vi "BCU诊断标定.vi"(8 "CAN端口":u16(ring) items=["0", "1"], 9 "设备索引号":u16(ring) items=["0", "1", "2", "3", "4", "5", "6", "7", "8", "9", "10", "11", "12", "13", "14", "15", ""], 10 "CAN卡类型":u32(ring)=21 items=["PCI5121"=1, "PCI9810"=2, "USBCAN1"=3, "USBCAN2"=4, "PCI9820"=5, "PCI5110"=7, "CANLite(mini)"=8, "ISA9620"=9, "ISA5420"=10, "PC104CAN"=11, "DNP9810"=13, "PCI9840B"=14, "PC104C2"=15, "PCI9820I"=16, "pec9920"=18, "USBCAN_E_U"=20, "USBCAN_2E_U"=21], 11 "Myindex":dbl=1.0) -> (3 "成功":bool)   [LabVIEW 2013]
uses:
  <vilib>/Utility/config.llb/Read Key (String).vi
  <vilib>/Utility/config.llb/Write Key (Path).vi
  <vilib>/Utility/file.llb/Write To Spreadsheet File (string).vi
  <vilib>/Utility/config.llb/Write Key (String).vi
  <vilib>/Utility/config.llb/NI_LVConfig.lvlib
  <vilib>/Utility/file.llb/Read From Spreadsheet File (string).vi
panel:
  out "读取超时":bool
  out "流控帧":bool
  out "流控帧 2":bool=TRUE
  in  "二维码 2":string="BNET01"
  out "失败?":bool=TRUE
  in  "主板选项":string(tree)="项目信息"
  out "重试次数":u8
  in  "模块版本读取":bool
  in  "模块软件版本":T1(ring)
  out "模块软件版本 2":i32(listbox)=-1
  out "从板信息":T2
  out "从板项目信息":bool
  out "项目信息结果":bool
  out "正级继电器 10":bool
  out "正级继电器 9":bool
  out "正级继电器 8":bool
  out "正级继电器 7":bool
  out "正级继电器 6":bool
  out "正级继电器 5":bool
  out "正级继电器 4":bool
  out "正级继电器 3":bool
  out "正级继电器 2":bool
  out "正级继电器 12":bool
  out "正级继电器 11":bool
  in  "DO1 2":bool
  out "模块个数":u8[](array[numeric])
  out "模块版本值":string[][](array[string])
  out "模块版本名称":string[][](array[string])
  out "硬件版本":string[](array[string])
  out "项目软件版本":string[](array[string])
  out "平台软件版本":string[](array[string])
  in  "读参数":T3
  out "MODEL号":u8[](array[numeric])
  out "主板数据":T4
  in  "布尔":bool=TRUE
  out "1 13":bool
  in  "error out":errorcluster
  out "key names":string[](array[string])
  out "输出数组":string[][](array[string])
  in  "当前从板板号":u8=1
  in  "高压参数":T5={"充电能量阀值"=375.0, "放电能量阀值"=375.0, "电流增益"=0.0, "平均电流"=0.0, "电压增益"=0.0, "平均电压"=0.0}
  in  "清BUFF":bool=TRUE
  out "继电器超时处理":bool
  in  "判定3":bool=TRUE
  out "判定2":bool
  in  "消除":bool
  in  "控制1":bool
  out "命令序号":u8=5
  in  "停止 2":bool
  in  "停止":bool
  in  "选项卡控件":enum32{"主板", "从板"}(tab)=enum."从板"
  in  "主板数据":string[][](table)=[["参数", "写入", "读取", "参数", "写入", "读取", "一级故障", "写入", "读取", "二级故障", "写入", "读取", "三张故障", "写入", "读取", "参数", "写入", "读取", "电池信息", "写入", "读取", "历史信息", "写入", "读取"], ["", "", "", "humd_sensr_no", "", "", "总电压过高", "", "", "总电压过高", "", "", "总电压过高", "", "", "风机开启温度", "", "", "电池串联数", "", "", "历史最高电压", "", ""], ["", "", "", "温度传感器类型", "", "", "总电压过低", "", "", "总电压过低", "", "", "总电压过低", "", "", "风机关闭温度", "", "", "电池并联数", "", "", "历史最低电压", "", ""], ["", "", "", "电流传感器类型", "", "", "温度过高", "", "", "温度过高", "", "", "温度过高", "", "", "加热开启温度", "", "", "电池厂商", "", "", "历史电池电压极差", "", ""], ["", "", "", "集成单板电压个数", "", "", "温度过低", "", "", "温度过低", "", "", "温度过低", "", "", "加热关闭温度", "", "", "电池类型", "", "", "历史最高平均电压", "", ""], ["", "", "", "集成单体温度个数", "", "", "整组温度不均衡", "", "", "整组温度不均衡", "", "", "整组温度不均衡", "", "", "风机开启温差", "", "", "年", "", "", "历史最低平均电压", "", ""], ["", "", "", "SOC", "", "", "单组电压不均衡", "", "", "单组电压不均衡", "", "", "单组电压不均衡", "", "", "风机关闭温差", "", "", "月", "", "", "历史最高端电压", "", ""], ["", "", "", "电池额定容量", "", "", "整组电压不均衡", "", "", "整组电压不均衡", "", "", "整组电压不均衡", "", "", "最大允许单体电压", "", "", "日", "", "", "历史最低端电压", "", ""], ["", "", "", "电池实际容量", "", "", "单体电压过高", "", "", "单体电压过高", "", "", "单体电压过高", "", "", "最大允许总电压", "", "", "电池包额定能量", "", "", "历史最高温度", "", ""], ["", "", "", "配置文件版本", "", "", "单体电压过低", "", "", "单体电压过低", "", "", "单体电压过低", "", "", "最大允许充电电流", "", "", "电池包额定容量", "", "", "历史最低温度", "", ""], ["", "", "", "车牌号", "", "", "充电电流过高", "", "", "充电电流过高", "", "", "充电电流过高", "", "", "最大允许温度", "", "", "电池包额定总电压", "", "", "历史电池温度极差", "", ""], ["", "", "", "从板板号", "", "", "放电电流过高", "", "", "放电电流过高", "", "", "放电电流过高", "", "", "最小充电电流", "", "", "电池包组号", "", "", "历史最高平均温度", "", ""], ["", "", "", "SOH", "", "", "单组温度不均衡", "", "", "单组温度不均衡", "", "", "单组温度不均衡", "", "", "电流步长", "", "", "电池包产权标识", "", "", "历史最低平均温度", "", ""], ["", "", "", "SOE", "", "", "SOC过高", "", "", "SOC过高", "", "", "SOC过高", "", "", "最小允许单体电压", "", "", "电池包应用车型", "", "", "平均温度分布", "", ""], ["", "", "", "产品编号", "", "", "SOC过低", "", "", "SOC过低", "", "", "SOC过低", "", "", "最大允许充电温度", "", "", "正极接触器寿命", "", "", "最低温度分布", "", ""], ["", "", "", "", "", "", "", "", "", "", "", "", "", "", "", "最小允许温度", "", "", "负极接触器寿命", "", "", "最高温度分布", "", ""], ["", "", "", "", "", "", "", "", "", "", "", "", "", "", "", "充电时间", "", "", "预充电接触器寿命", "", "", "最大极差温度分布", "", ""], ["", "", "", "", "", "", "", "", "", "", "", "", "", "", "", "", "", "", "充电接触器寿命", "", "", "历史最大充电功率", "", ""], ["", "", "", "", "", "", "", "", "", "", "", "", "", "", "", "", "", "", "车辆VIN号", "", "", "历史最大放电功率", "", ""], ["", "", "", "", "", "", "", "", "", "", "", "", "", "", "", "", "", "", "电池放空次数", "", "", "历史最大充电电流", "", ""], ["", "", "", "", "", "", "", "", "", "", "", "", "", "", "", "", "", "", "充满次数", "", "", "历史最大放电电流", "", ""], ["", "", "", "", "", "", "", "", "", "", "", "", "", "", "", "", "", "", "充电次数", "", "", "电池组工作电流分布", "", ""], ["", "", "", "", "", "", "", "", "", "", "", "", "", "", "", "", "", "", "", "", "", "电池组SOC分布", "", ""], ["", "", "", "", "", "", "", "", "", "", "", "", "", "", "", "", "", "", "", "", "", "电池总充电安时", "", ""], ["", "", "", "", "", "", "", "", "", "", "", "", "", "", "", "", "", "", "", "", "", "电池总放电安时", "", ""], ["", "", "", "", "", "", "", "", "", "", "", "", "", "", "", "", "", "", "", "", "", "电池剩余容量", "", ""], ["", "", "", "", "", "", "", "", "", "", "", "", "", "", "", "", "", "", "", "", "", "", "", ""], ["", "", "", "", "", "", "", "", "", "", "", "", "", "", "", "", "", "", "", "", "", "", "", ""], ["", "", "", "", "", "", "", "", "", "", "", "", "", "", "", "", "", "", "", "", "", "", "", ""], ["", "", "", "", "", "", "", "", "", "", "", "", "", "", "", "", "", "", "", "", "", "", "", ""], ["", "", "", "", "", "", "", "", "", "", "", "", "", "", "", "", "", "", "", "", "", "", "", ""], ["", "", "", "", "", "", "", "", "", "", "", "", "", "", "", "", "", "", "", "", "", "", "", ""], ["", "", "", "", "", "", "", "", "", "", "", "", "", "", "", "", "", "", "", "", "", "", "", ""], ["", "", "", "", "", "", "", "", "", "", "", "", "", "", "", "", "", "", "", "", "", "", "", ""], ["", "", "", "", "", "", "", "", "", "", "", "", "", "", "", "", "", "", "", "", "", "", "", ""], ["", "", "", "", "", "", "", "", "", "", "", "", "", "", "", "", "", "", "", "", "", "", "", ""], ["", "", "", "", "", "", "", "", "", "", "", "", "", "", "", "", "", "", "", "", "", "", "", ""], ["", "", "", "", "", "", "", "", "", "", "", "", "", "", "", "", "", "", "", "", "", "", "", ""], ["", "", "", "", "", "", "", "", "", "", "", "", "", "", "", "", "", "", "", "", "", "", "", ""], ["", "", "", "", "", "", "", "", "", "", "", "", "", "", "", "", "", "", "", "", "", "", "", ""], ["", "", "", "", "", "", "", "", "", "", "", "", "", "", "", "", "", "", "", "", "", "", "", ""], ["", "", "", "", "", "", "", "", "", "", "", "", "", "", "", "", "", "", "", "", "", "", "", ""], ["", "", "", "", "", "", "", "", "", "", "", "", "", "", "", "", "", "", "", "", "", "", "", ""], ["", "", "", "", "", "", "", "", "", "", "", "", "", "", "", "", "", "", "", "", "", "", "", ""], ["", "", "", "", "", "", "", "", "", "", "", "", "", "", "", "", "", "", "", "", "", "", "", ""], ["", "", "", "", "", "", "", "", "", "", "", "", "", "", "", "", "", "", "", "", "", "", "", ""], ["", "", "", "", "", "", "", "", "", "", "", "", "", "", "", "", "", "", "", "", "", "", "", ""], ["", "", "", "", "", "", "", "", "", "", "", "", "", "", "", "", "", "", "", "", "", "", "", ""], ["", "", "", "", "", "", "", "", "", "", "", "", "", "", "", "", "", "", "", "", "", "", "", ""], ["", "", "", "", "", "", "", "", "", "", "", "", "", "", "", "", "", "", "", "", "", "", "", ""], ["", "", "", "", "", "", "", "", "", "", "", "", "", "", "", "", "", "", "", "", "", "", "", ""], ["", "", "", "", "", "", "", "", "", "", "", "", "", "", "", "", "", "", "", "", "", "", "", ""], ["", "", "", "", "", "", "", "", "", "", "", "", "", "", "", "", "", "", "", "", "", "", "", ""], ["", "", "", "", "", "", "", "", "", "", "", "", "", "", "", "", "", "", "", "", "", "", "", ""], ["", "", "", "", "", "", "", "", "", "", "", "", "", "", "", "", "", "", "", "", "", "", "", ""], ["", "", "", "", "", "", "", "", "", "", "", "", "", "", "", "", "", "", "", "", "", "", "", ""], ["", "", "", "", "", "", "", "", "", "", "", "", "", "", "", "", "", "", "", "", "", "", "", ""], ["", "", "", "", "", "", "", "", "", "", "", "", "", "", "", "", "", "", "", "", "", "", "", ""], ["", "", "", "", "", "", "", "", "", "", "", "", "", "", "", "", "", "", "", "", "", "", "", ""], ["", "", "", "", "", "", "", "", "", "", "", "", "", "", "", "", "", "", "", "", "", "", "", ""], ["", "", "", "", "", "", "", "", "", "", "", "", "", "", "", "", "", "", "", "", "", "", "", ""], ["", "", "", "", "", "", "", "", "", "", "", "", "", "", "", "", "", "", "", "", "", "", "", ""], ["", "", "", "", "", "", "", "", "", "", "", "", "", "", "", "", "", "", "", "", "", "", "", ""], ["", "", "", "", "", "", "", "", "", "", "", "", "", "", "", "", "", "", "", "", "", "", "", ""], ["", "", "", "", "", "", "", "", "", "", "", "", "", "", "", "", "", "", "", "", "", "", "", ""], ["", "", "", "", "", "", "", "", "", "", "", "", "", "", "", "", "", "", "", "", "", "", "", ""], ["", "", "", "", "", "", "", "", "", "", "", "", "", "", "", "", "", "", "", "", "", "", "", ""], ["", "", "", "", "", "", "", "", "", "", "", "", "", "", "", "", "", "", "", "", "", "", "", ""], ["", "", "", "", "", "", "", "", "", "", "", "", "", "", "", "", "", "", "", "", "", "", "", ""], ["", "", "", "", "", "", "", "", "", "", "", "", "", "", "", "", "", "", "", "", "", "", "", ""], ["", "", "", "", "", "", "", "", "", "", "", "", "", "", "", "", "", "", "", "", "", "", "", ""], ["", "", "", "", "", "", "", "", "", "", "", "", "", "", "", "", "", "", "", "", "", "", "", ""], ["", "", "", "", "", "", "", "", "", "", "", "", "", "", "", "", "", "", "", "", "", "", "", ""], ["", "", "", "", "", "", "", "", "", "", "", "", "", "", "", "", "", "", "", "", "", "", "", ""], ["", "", "", "", "", "", "", "", "", "", "", "", "", "", "", "", "", "", "", "", "", "", "", ""], ["", "", "", "", "", "", "", "", "", "", "", "", "", "", "", "", "", "", "", "", "", "", "", ""], ["", "", "", "", "", "", "", "", "", "", "", "", "", "", "", "", "", "", "", "", "", "", "", ""], ["", "", "", "", "", "", "", "", "", "", "", "", "", "", "", "", "", "", "", "", "", "", "", ""], ["", "", "", "", "", "", "", "", "", "", "", "", "", "", "", "", "", "", "", "", "", "", "", ""], ["", "", "", "", "", "", "", "", "", "", "", "", "", "", "", "", "", "", "", "", "", "", "", ""], ["", "", "", "", "", "", "", "", "", "", "", "", "", "", "", "", "", "", "", "", "", "", "", ""], ["", "", "", "", "", "", "", "", "", "", "", "", "", "", "", "", "", "", "", "", "", "", "", ""], ["", "", "", "", "", "", "", "", "", "", "", "", "", "", "", "", "", "", "", "", "", "", "", ""], ["", "", "", "", "", "", "", "", "", "", "", "", "", "", "", "", "", "", "", "", "", "", "", ""], ["", "", "", "", "", "", "", "", "", "", "", "", "", "", "", "", "", "", "", "", "", "", "", ""], ["", "", "", "", "", "", "", "", "", "", "", "", "", "", "", "", "", "", "", "", "", "", "", ""], ["", "", "", "", "", "", "", "", "", "", "", "", "", "", "", "", "", "", "", "", "", "", "", ""], ["", "", "", "", "", "", "", "", "", "", "", "", "", "", "", "", "", "", "", "", "", "", "", ""], ["", "", "", "", "", "", "", "", "", "", "", "", "", "", "", "", "", "", "", "", "", "", "", ""], ["", "", "", "", "", "", "", "", "", "", "", "", "", "", "", "", "", "", "", "", "", "", "", ""], ["", "", "", "", "", "", "", "", "", "", "", "", "", "", "", "", "", "", "", "", "", "", "", ""], ["", "", "", "", "", "", "", "", "", "", "", "", "", "", "", "", "", "", "", "", "", "", "", ""], ["", "", "", "", "", "", "", "", "", "", "", "", "", "", "", "", "", "", "", "", "", "", "", ""], ["", "", "", "", "", "", "", "", "", "", "", "", "", "", "", "", "", "", "", "", "", "", "", ""], ["", "", "", "", "", "", "", "", "", "", "", "", "", "", "", "", "", "", "", "", "", "", "", ""], ["", "", "", "", "", "", "", "", "", "", "", "", "", "", "", "", "", "", "", "", "", "", "", ""], ["", "", "", "", "", "", "", "", "", "", "", "", "", "", "", "", "", "", "", "", "", "", "", ""], ["", "", "", "", "", "", "", "", "", "", "", "", "", "", "", "", "", "", "", "", "", "", "", ""], ["", "", "", "", "", "", "", "", "", "", "", "", "", "", "", "", "", "", "", "", "", "", "", ""], ["", "", "", "", "", "", "", "", "", "", "", "", "", "", "", "", "", "", "", "", "", "", "", ""], ["", "", "", "", "", "", "", "", "", "", "", "", "", "", "", "", "", "", "", "", "", "", "", ""], [" ", "", "", "", "", "", "", "", "", "", "", "", "", "", "", "", "", "", "", "", "", "", "", ""]] caption="故障阀值信息"
  in  "从板表格":string[][](table)=[["参数", "写入", "读取", "参数", "写入", "读取", "二级故障参数", "写入", "读取", "快换参数", "写入", "读取", "快换参数", "写入", "读取"], ["", "", "", "", "", "", "电压过高", "", "", "电池类型", "", "", "最大允许单体电压", "", ""], ["", "", "", "风机开启温度", "", "", "电压过低", "", "", "电池厂家", "", "", "最大允许总电压", "", ""], ["", "", "", "风机关闭温度", "", "", "电压不均衡", "", "", "年", "", "", "最大允许温度", "", ""], ["", "", "", "加热开启温度", "", "", "温度过高", "", "", "月", "", "", "最小允许温度", "", ""], ["", "", "", "加热关闭温度", "", "", "温度过低", "", "", "日", "", "", "最大允许电流", "", ""], ["", "", "", "风机开启温差", "", "", "温度不均衡", "", "", "运行模式", "", "", "车牌号", "", ""], ["", "", "", "风机关闭温差", "", "", "容量不均衡", "", "", "从板号", "", "", "SOC", "", ""], ["", "", "", "一级故障参数", "", "", "三级故障参数", "", "", "电池地区", "", "", "安时数", "", ""], ["", "", "", "电压过高", "", "", "电压过高", "", "", "电池组序号", "", "", "充电总安时", "", ""], ["", "", "", "电压过低", "", "", "电压过低", "", "", "电池包串联数", "", "", "放电总安时", "", ""], ["", "", "", "电压不均衡", "", "", "电压不均衡", "", "", "电池包并联数", "", "", "", "", ""], ["", "", "", "温度过高", "", "", "温度过高", "", "", "电池包安时数", "", "", "", "", ""], ["", "", "", "温度过低", "", "", "温度过低", "", "", "充电次数", "", "", "", "", ""], ["", "", "", "温度不均衡", "", "", "温度不均衡", "", "", "", "", "", "", "", ""], ["", "", "", "容量不均衡", "", "", "容量不均衡", "", "", "", "", "", "", "", ""], ["", "", "", "", "", "", "", "", "", "", "", "", "", "", ""], ["", "", "", "", "", "", "", "", "", "", "", "", "", "", ""], ["", "", "", "", "", "", "", "", "", "", "", "", "", "", ""], ["", "", "", "", "", "", "", "", "", "", "", "", "", "", ""], ["", "", "", "", "", "", "", "", "", "", "", "", "", "", ""], ["", "", "", "", "", "", "", "", "", "", "", "", "", "", ""], ["", "", "", "", "", "", "", "", "", "", "", "", "", "", ""], ["", "", "", "", "", "", "", "", "", "", "", "", "", "", ""], ["", "", "", "", "", "", "", "", "", "", "", "", "", "", ""], ["", "", "", "", "", "", "", "", "", "", "", "", "", "", ""], ["", "", "", "", "", "", "", "", "", "", "", "", "", "", ""], ["", "", "", "", "", "", "", "", "", "", "", "", "", "", ""], ["", "", "", "", "", "", "", "", "", "", "", "", "", "", ""], ["", "", "", "", "", "", "", "", "", "", "", "", "", "", ""], ["", "", "", "", "", "", "", "", "", "", "", "", "", "", ""], ["", "", "", "", "", "", "", "", "", "", "", "", "", "", ""], ["", "", "", "", "", "", "", "", "", "", "", "", "", "", ""], ["", "", "", "", "", "", "", "", "", "", "", "", "", "", ""], ["", "", "", "", "", "", "", "", "", "", "", "", "", "", ""], ["", "", "", "", "", "", "", "", "", "", "", "", "", "", ""], ["", "", "", "", "", "", "", "", "", "", "", "", "", "", ""], ["", "", "", "", "", "", "", "", "", "", "", "", "", "", ""], ["", "", "", "", "", "", "", "", "", "", "", "", "", "", ""], ["", "", "", "", "", "", "", "", "", "", "", "", "", "", ""], ["", "", "", "", "", "", "", "", "", "", "", "", "", "", ""], ["", "", "", "", "", "", "", "", "", "", "", "", "", "", ""], ["", "", "", "", "", "", "", "", "", "", "", "", "", "", ""], ["", "", "", "", "", "", "", "", "", "", "", "", "", "", ""], ["", "", "", "", "", "", "", "", "", "", "", "", "", "", ""], ["", "", "", "", "", "", "", "", "", "", "", "", "", "", ""], ["", "", "", "", "", "", "", "", "", "", "", "", "", "", ""], ["", "", "", "", "", "", "", "", "", "", "", "", "", "", ""], ["", "", "", "", "", "", "", "", "", "", "", "", "", "", ""], ["", "", "", "", "", "", "", "", "", "", "", "", "", "", ""], ["", "", "", "", "", "", "", "", "", "", "", "", "", "", ""], ["", "", "", "", "", "", "", "", "", "", "", "", "", "", ""], ["", "", "", "", "", "", "", "", "", "", "", "", "", "", ""], ["", "", "", "", "", "", "", "", "", "", "", "", "", "", ""], ["", "", "", "", "", "", "", "", "", "", "", "", "", "", ""], ["", "", "", "", "", "", "", "", "", "", "", "", "", "", ""], ["", "", "", "", "", "", "", "", "", "", "", "", "", "", ""], ["", "", "", "", "", "", "", "", "", "", "", "", "", "", ""], ["", "", "", "", "", "", "", "", "", "", "", "", "", "", ""], ["", "", "", "", "", "", "", "", "", "", "", "", "", "", ""], ["", "", "", "", "", "", "", "", "", "", "", "", "", "", ""], ["", "", "", "", "", "", "", "", "", "", "", "", "", "", ""], ["", "", "", "", "", "", "", "", "", "", "", "", "", "", ""], ["", "", "", "", "", "", "", "", "", "", "", "", "", "", ""], ["", "", "", "", "", "", "", "", "", "", "", "", "", "", ""], ["", "", "", "", "", "", "", "", "", "", "", "", "", "", ""], ["", "", "", "", "", "", "", "", "", "", "", "", "", "", ""], ["", "", "", "", "", "", "", "", "", "", "", "", "", "", ""], ["", "", "", "", "", "", "", "", "", "", "", "", "", "", ""], ["", "", "", "", "", "", "", "", "", "", "", "", "", "", ""], ["", "", "", "", "", "", "", "", "", "", "", "", "", "", ""], ["", "", "", "", "", "", "", "", "", "", "", "", "", "", ""], ["", "", "", "", "", "", "", "", "", "", "", "", "", "", ""], ["", "", "", "", "", "", "", "", "", "", "", "", "", "", ""], ["", "", "", "", "", "", "", "", "", "", "", "", "", "", ""], ["", "", "", "", "", "", "", "", "", "", "", "", "", "", ""], ["", "", "", "", "", "", "", "", "", "", "", "", "", "", ""], ["", "", "", "", "", "", "", "", "", "", "", "", "", "", ""], ["", "", "", "", "", "", "", "", "", "", "", "", "", "", ""], ["", "", "", "", "", "", "", "", "", "", "", "", "", "", ""], ["", "", "", "", "", "", "", "", "", "", "", "", "", "", ""], ["", "", "", "", "", "", "", "", "", "", "", "", "", "", ""], ["", "", "", "", "", "", "", "", "", "", "", "", "", "", ""], ["", "", "", "", "", "", "", "", "", "", "", "", "", "", ""], ["", "", "", "", "", "", "", "", "", "", "", "", "", "", ""], ["", "", "", "", "", "", "", "", "", "", "", "", "", "", ""], ["", "", "", "", "", "", "", "", "", "", "", "", "", "", ""], ["", "", "", "", "", "", "", "", "", "", "", "", "", "", ""], ["", "", "", "", "", "", "", "", "", "", "", "", "", "", ""], ["", "", "", "", "", "", "", "", "", "", "", "", "", "", ""], ["", "", "", "", "", "", "", "", "", "", "", "", "", "", ""], ["", "", "", "", "", "", "", "", "", "", "", "", "", "", ""], ["", "", "", "", "", "", "", "", "", "", "", "", "", "", ""], ["", "", "", "", "", "", "", "", "", "", "", "", "", "", ""], ["", "", "", "", "", "", "", "", "", "", "", "", "", "", ""], ["", "", "", "", "", "", "", "", "", "", "", "", "", "", ""], ["", "", "", "", "", "", "", "", "", "", "", "", "", "", ""], ["", "", "", "", "", "", "", "", "", "", "", "", "", "", ""], ["", "", "", "", "", "", "", "", "", "", "", "", "", "", ""], ["", "", "", "", "", "", "", "", "", "", "", "", "", "", ""], ["", "", "", "", "", "", "", "", "", "", "", "", "", "", ""], [" ", "", "", "", "", "", "", "", "", "", "", "", "", "", ""]]
  in  "读取转换为写入":bool
  in  "主界面选项":enum32{"单选选项1", "单选选项2", "单选选项2 2", "单选选项2 3"}(radio)
  in  "命令":u8=133 format="%x"
  in  "写?":bool
  in  "VCI_Receive":T6 {"Rsv3" max=0 format="%x"; "Rsv2" min=101 format="%x"; "Rsv1" format="%x"; "Data8" format="%x"; "Data7" format="%x"; "Data6" format="%x"; "Data5" format="%x"; "Data4" format="%x"; "Data3" format="%x"; "Data2" format="%x"; "Data1" format="%x"; "DataLen" format="%x"; "ExternFlag" format="%x"; "RemoteFlag" format="%x"; "SendType" format="%x"; "TimeFlag" format="%x"; "TimeStamp" format="%x"; "ID" format="%x"}
  in  "面板选择":T7(tab)
  in  "终止读写按钮":bool
  in  "路径":path
  in  "强制终止读写标记":bool
  in  "从板选项":string(tree)="从板信息"
  in  "主从选择":enum32{"主板", "从板"}(tab)
  in  "1 11":bool
  in  "1 5":bool
  in  "1 4":bool
  in  "1 3":bool
  in  "1 2":bool
  in  "1":bool=TRUE
  in  "主板2":T8(tab)
  in  "二维码":string="BNET01"
  in  "项目信息":string[][](table)=[["主板电池节数", "36"], ["从板1电池节数", "36"], ["第1通道电压个数", "12"], ["第2通道电压个数", "12"], ["第3通道电压个数", "12"], ["第4通道电压个数", "0"], ["第5通道电压个数", "0"], ["第6通道电压个数", "0"], ["第7通道电压个数", "0"], ["第8通道电压个数", "0"], ["第9通道电压个数", "0"], ["第10通道电压个数", "0"], ["第11通道电压个数", "0"], ["第12通道电压个数", "0"], ["第13通道电压个数", "0"], ["第14通道电压个数", "0"], ["第15通道电压个数", "0"], ["第16通道电压个数", "0"], ["第17通道电压个数", "0"], ["第18通道电压个数", "0"], ["第19通道电压个数", "0"], ["第20通道电压个数", "0"], ["主板电压起始值", "1"], ["从板1电压起始值", "1"], ["主板温度个数", "8"], ["从板1温度个数", "8"], ["主板温度起始值", "1"], ["从板1温度起始值", "1"], ["第一个保险通道", "0"], ["第一个保险位置", "0"], ["第二个保险通道", "0"], ["第二个保险位置", "0"], ["第三个保险通道", "0"], ["第三个保险位置", "0"], ["第四个保险通道", ""], ["第四个保险位置", ""], ["第五个保险通道", ""], ["第五个保险位置", ""], ["第六个保险通道", ""], ["第六个保险位置", ""], ["第七个保险通道", ""], ["第七个保险位置", ""], ["第八个保险通道", ""], ["第八个保险位置", ""], ["第九个保险通道", ""], ["第九个保险位置", ""], ["第十个保险通道", ""], ["第十个保险位置", ""]]
  in  "项目信息2":T9={"电池额定容量(A)"=50.0, "使用者"=1.0, "电池实际容量(A)"=50.0, "车架(牌)号"="0000001", "配置文件版本"="BNET01", "SOH(%)"=100.0, "SOC(%)"=100.0, "产品编号"="000001", "系统时钟"="2014-03-28 18:22:37"} caption="项目信息二"
  in  "一级故障":T10={"总电压过高"=389.0, "整组电压不均衡"=0.5, "SOC过高"=101.0, "单体电压过高"=4.23, "总电压过低"=276.0, "温度过高"=50.0, "温度过低"=-20.0, "单组电压不均衡"=0.5, "整组温度不均衡"=25.0, "单组温度不均衡"=25.0, "单体电压过低"=3.0, "充电电流过高"=110.0, "放电电流过高"=250.0, "SOC过低"=30.0, "内阻过大"=3.0, "极柱温度过高"=50.0, "SOH过低"=90.0}
  in  "一级故障 2":T10={"总电压过高"=391.0, "整组电压不均衡"=1.0, "SOC过高"=101.0, "单体电压过高"=4.25, "总电压过低"=253.0, "温度过高"=55.0, "温度过低"=-30.0, "单组电压不均衡"=1.0, "整组温度不均衡"=30.0, "单组温度不均衡"=30.0, "单体电压过低"=2.75, "充电电流过高"=132.0, "放电电流过高"=270.0, "SOC过低"=20.0, "内阻过大"=5.0, "极柱温度过高"=55.0, "SOH过低"=80.0} caption="二级故障"
  in  "一级故障 3":T10={"总电压过高"=395.0, "整组电压不均衡"=1.5, "SOC过高"=101.0, "单体电压过高"=4.3, "总电压过低"=230.0, "温度过高"=60.0, "温度过低"=-40.0, "单组电压不均衡"=1.5, "整组温度不均衡"=35.0, "单组温度不均衡"=35.0, "单体电压过低"=2.5, "充电电流过高"=165.0, "放电电流过高"=300.0, "SOC过低"=10.0, "内阻过大"=10.0, "极柱温度过高"=60.0, "SOH过低"=70.0} caption="三级故障"
  in  "加热控制参数":T11={"风机开启温度"=30.0, "风机关闭温度"=20.0, "加热开启温度"=10.0, "加热关闭温度"=15.0, "风机开启温差"=5.0, "风机关闭温差"=3.0, "加热关闭温差"=10.0}
  in  "一级故障 5":T12={"最大允许单体电压"=3.7, "最大允许总电压"=365.0, "最小允许单体电压"=2.8, "最大允许充电电流"=400.0, "最小允许充电电流"=100.0, "最大允许充电温度"=50.0, "最小允许充电温度"=10.0, "电流步长"=5.0} caption="充电控制参数"
  in  "电池信息":T13={"电池串联"=92.0, "电池并联"=2.0, "累计放电总安时"=0.0, "电池包额定容量"=67.0, "电池包额定能量(kWh)"=0.0, "电池包额定总电压"=340.0, "累计充电总安时"=0.0, "电池充满次数"=0.0, "电池放空次数"=0.0, "电池充电次数"=0.0, "电池生产日期"="2013-12-11 11:34:30", "电池厂家"="普莱德", "电池类型"="磷酸铁锂", "电池包组号"="0", "电池包产权标识"="122", "电池应用车型"="123", "实际容量"=67.0}
  in  "1 10":bool
  in  "1 9":bool
  in  "1 8":bool
  in  "1 7":bool
  in  "1 6":bool
  in  "1 12":bool
  in  "等级 2":T14(tab)
  in  "加热控制参数":T11={"风机开启温度"=30.0, "风机关闭温度"=20.0, "加热开启温度"=10.0, "加热关闭温度"=15.0, "风机开启温差"=5.0, "风机关闭温差"=3.0, "加热关闭温差"=15.0}
  in  "项目信息 2":string[][](table)=[["电压个数", "32"], ["电压起始值", "33"], ["第1通道电压个数", "8"], ["第2通道电压个数", "12"], ["第3通道电压个数", "12"], ["第4通道电压个数", "0"], ["第5通道电压个数", "0"], ["第6通道电压个数", "0"], ["第7通道电压个数", "0"], ["第8通道电压个数", "0"], ["第9通道电压个数", "0"], ["第10通道电压个数", "0"], ["第11通道电压个数", ""], ["第12通道电压个数", ""], ["第13通道电压个数", ""], ["第14通道电压个数", ""], ["第15通道电压个数", ""], ["第16通道电压个数", ""], ["第17通道电压个数", ""], ["第18通道电压个数", ""], ["第19通道电压个数", ""], ["第20通道电压个数", ""], ["温度个数", "8"], ["温度起始值", "7"], ["第一个保险通道", "1"], ["第一个保险位置", "5"], ["第二个保险通道", ""], ["第二个保险位置", ""], ["第三个保险通道", ""], ["第三个保险位置", ""], ["第四个保险通道", ""], ["第四个保险位置", ""], ["第五个保险通道", ""], ["第五个保险位置", ""], ["第六个保险通道", ""], ["第六个保险位置", ""], ["第七个保险通道", ""], ["第七个保险位置", ""], ["第八个保险通道", ""], ["第八个保险位置", ""], ["第九个保险通道", ""], ["第九个保险位置", ""], ["第十个保险通道", ""], ["第十个保险位置", ""], ["", ""], ["", ""], ["", ""], ["", ""], ["", ""], ["", ""], ["", ""], ["", ""], ["", ""], ["", ""], ["", ""], ["", ""], ["", ""], ["", ""], ["", ""], ["", ""], ["", ""], ["", ""], ["", ""], ["", ""], ["", ""], ["", ""], ["", ""], ["", ""], ["", ""], ["", ""], ["", ""], ["", ""], ["", ""], ["", ""], ["", ""], ["", ""], ["", ""], ["", ""], ["", ""], ["", ""], ["", ""], ["", ""], ["", ""], ["", ""]]
  in  "一级故障 6":T15={"电压过高"=4.0, "电压过低"=3.5, "温度过高"=50.0, "温度过低"=0.0, "电压不均衡(V)"=0.3, "温度不均衡"=10.0, "SOC过低"=10.0} caption="一级故障"
  in  "一级故障 7":T15={"电压过高"=4.1, "电压过低"=3.3, "温度过高"=55.0, "温度过低"=-5.0, "电压不均衡(V)"=0.4, "温度不均衡"=10.0, "SOC过低"=5.0} caption="二级故障"
  in  "一级故障 8":T15={"电压过高"=4.2, "电压过低"=3.2, "温度过高"=60.0, "温度过低"=-10.0, "电压不均衡(V)"=0.5, "温度不均衡"=15.0, "SOC过低"=0.0} caption="三级故障"
  in  "快换":bool caption="快换写入"
  in  "电池组信息":T16
  in  "均衡参数":T17 {"充电结束电压(100%)" min=0 max=5 format="%#.4f"; "充电结束电压(99%)" min=0 max=5 format="%#.4f"; "充电结束电压(98%)" min=0 max=5 format="%#.4f"; "充电结束电压(97%)" min=0 max=5 format="%#.4f"; "充电结束电压(96%)" min=0 max=5 format="%#.4f"; "充电结束电压(95%)" min=0 max=5 format="%#.4f"; "均衡计算-电压极差阀值" min=0 max=5 format="%#.4f"; "均衡停止-最低电压阀值" min=0 max=5 format="%#.4f"; "均衡计算-最低电压阀值" min=0 max=5 format="%#.4f"; "均衡计算-电压低阀值2级" min=0 max=5 format="%#.4f"; "充电结束电压(94%)" min=0 max=5 format="%#.4f"; "充电结束电压(93%)" min=0 max=5 format="%#.4f"; "均衡计算-电压低阀值1级" min=0 max=5 format="%#.4f"; "均衡计算-电压高阀值1级" min=0 max=5 format="%#.4f"; "均衡计算-电压高阀值2级" min=0 max=5 format="%#.4f"; "充电结束电压(92%)" min=0 max=5 format="%#.4f"; "充电结束电压(91%)" min=0 max=5 format="%#.4f"; "充电结束电压(90%)" min=0 max=5 format="%#.4f"}
  in  "主从板":enum32{"单选选项2", "单选选项1"}(radio)=enum."单选选项1"
  in  "读配置文件":bool
  in  "单个写入":bool
  in  "全部写入":bool
  in  "全部读取":bool
  in  "单个读取":bool
  in  "从板个数":dbl=1.0
  in  "结果":i32(listbox)=-1
  in  "保存主板参数":bool
  in  "从板号":u8=1 min=1 max=30
  out "CAN":bool=TRUE
  out "硬件版本号":string
  in  "保存版本信息":bool
  in  "强制停止版本读取":bool
  in  "从板板号":u8 caption="板号" max=30
  in  "结果":i32(listbox)=-1
  in  "项目软本读取":bool
  out "项目软件版本号":string
  out "平台软件版本号":string
  in  "平台软件版本读取":bool
  in  "读硬件版本号":bool
  in  "均衡屏":enum32{"选项卡 1"}(tab)
  in  "开启均衡":bool
  in  "DO屏":enum32{"选项卡 1"}(tab)
  in  "继电器屏1 2":enum32{"选项卡 1"}(tab)
  in  "继电器屏1 2":enum32{"选项卡 1"}(tab)
  in  "强制类型":enum16{"全通道开启", "单通道开启", "清待均衡时间"}(ring)
  in  "均衡类型选择":enum16{"放电均衡", "充电均衡", "充放电均衡"}(ring)
  in  "强制开启均衡":bool
  in  "关闭均衡":bool
  in  "控制按键全为关":bool
  in  "控制按键全为开":bool
  in  "DO2":bool
  in  "DO1":bool
  in  "动作保持时间":dbl
  in  "从板板号":u8=1 min=1 max=30
  in  "风机继电器(从)":bool caption="风机继电器"
  in  "加热继电器(从)":bool
  in  "风机继电器":bool
  in  "充电继电器":bool
  in  "加热继电器":bool
  in  "预充电继电器":bool
  in  "负级继电器":bool
  in  "正级继电器":bool
  in  "继电器全关":bool
  in  "继电器全开":bool
  in  "均衡位置":u16=1 min=1 max=400
  in  "均衡时间":dbl=20.0 min=0.0 max=5000.0 format="%#_6f"
  in  "从板板号 2":u8 caption="板号" max=30
  in  "状态选择":T18(ring)=enum."RS485,RS232检测故障"
  in  "读取故障详细状态":bool
  out "电池故障":string[][](array[string])
  in  "板类型":enum16{"集中式", "高压板"}(ring)
  in  "结果2":i32(listbox)
  # "从板"
  # "一级故障阀值"
  # "一级故障阀值"
  # "一级故障阀值"
  # "BCU参数设置"
  # "从\n    板"
  # "充电信息"
  # "\"0\"为主板"
  # "ms"
  # "继电器控制"
  # "主板"
  # "DO控制"
  # "主板"
  # "均衡控制"
  # "从板"
  # "继电器控制"
  # "从板"
  # "min"
  # "\"0\"为主板"
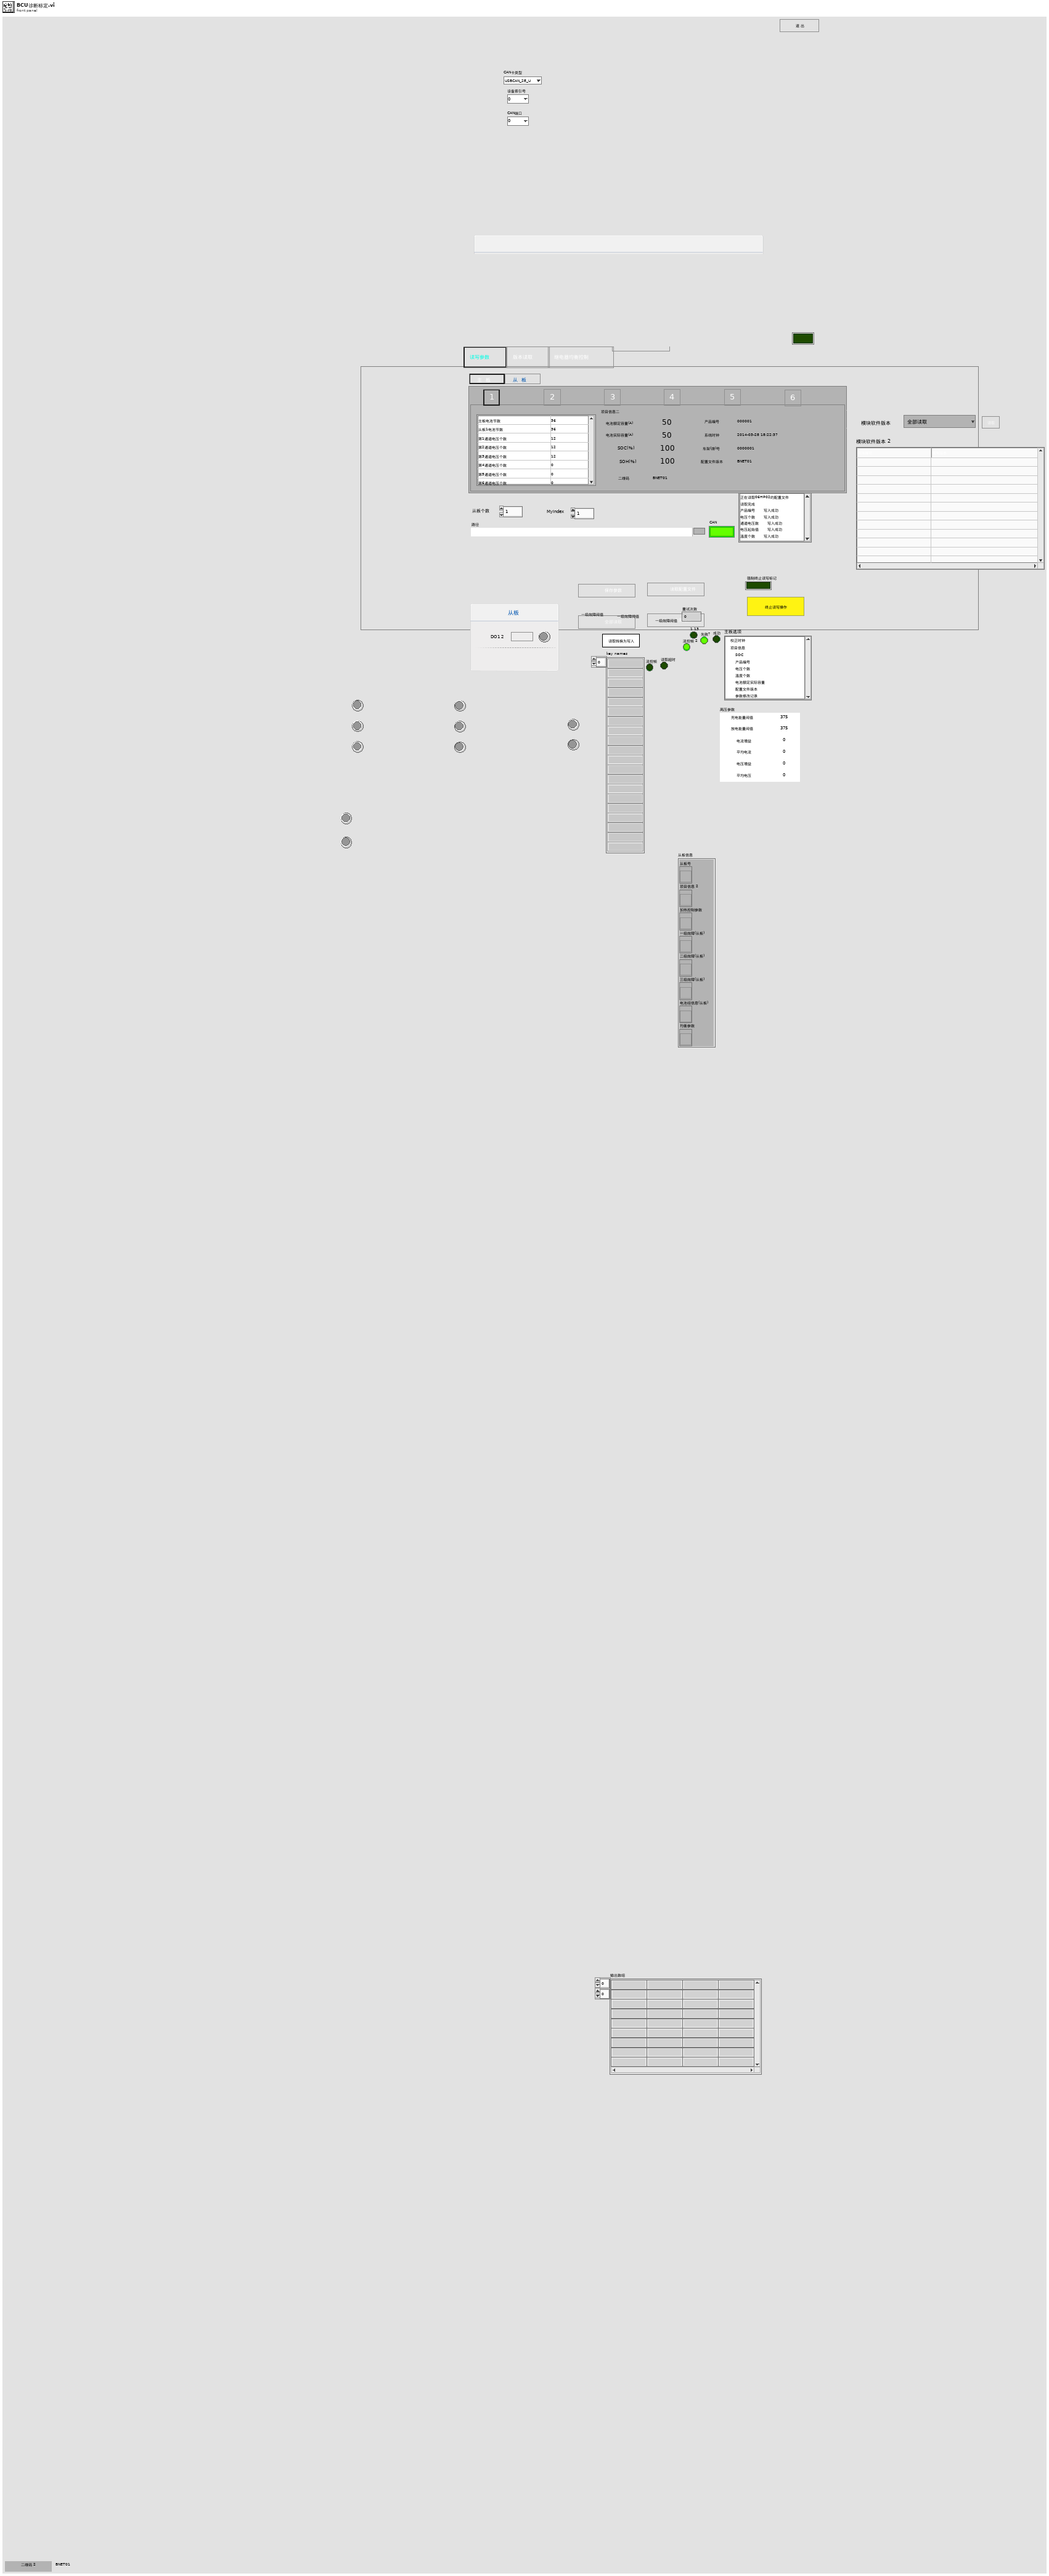
[diagram p1: front panel]
types:
  T1 = enum16{"全部读取", "VERSIONM", "BCUMCAL", "BMUMCAL", "BMURMCAL", "BCUCMCAL", "BCUDMCAL", "SCH", "BSW", "CDD", "DATALAYER", "DATAANALYSIS", "SOC", "SOH", "SOF", "INTRES", "INTCAN", "CARCAN", "CHGCANL", "THM", "CHGM", "HVM", "LVM", "BALM", "SAFEM", "RUNMODEM", "RALAY", "DO", "GBCHGDET", "SUPPLYPOWGDET", "SUMVDET", "CURDET", "TEMPERDET", "CELLVDET", "ISODET", "AI", "DI", "SYSCONF", "ECUCONF"}
  T2 = cluster{"从板号":refnum<vi>, "项目信息 2":refnum<vi>, "加热控制参数":refnum<vi>, "一级故障(从板)":refnum<vi>, "二级故障(从板)":refnum<vi>, "三级故障(从板)":refnum<vi>, "电池组信息(从板)":refnum<vi>, "均衡参数":refnum<vi>}
  T3 = cluster{"return type":u32, "pReceive":cluster{"ID":u32, "TimeStamp":u32, "TimeFlag":u8, "SendType":u8, "RemoteFlag":u8, "ExternFlag":u8, "DataLen":u8, u8, u8, u8, u8, u8, u8, u8, u8, u8, u8, u8}[]}
  T4 = cluster{"项目信息":refnum<vi>, "一级故障 4":refnum<vi>, "一级故障":refnum<vi>, "一级故障 2":refnum<vi>, "一级故障 3":refnum<vi>, "加热控制参数":refnum<vi>, "充电控制参数":refnum<vi>, "高压参数":refnum<vi>, "电池信息":refnum<vi>}
  T5 = cluster{"充电能量阀值":dbl, "放电能量阀值":dbl, "电流增益":dbl, "平均电流":dbl, "电压增益":dbl, "平均电压":dbl}
  T6 = cluster{"ID":u32, "TimeStamp":u32, "TimeFlag":u8, "SendType":u8, "RemoteFlag":u8, "ExternFlag":u8, "DataLen":u8, "Data1":u8, "Data2":u8, "Data3":u8, "Data4":u8, "Data5":u8, "Data6":u8, "Data7":u8, "Data8":u8, "Rsv1":u8, "Rsv2":u8, "Rsv3":u8}
  T7 = enum32{"读写参数", "版本读取", "其它诊断", "高压板校正", "高压板校正2"}
  T8 = enum32{"项目信息", "一级故障阀值", "二级故障阀值", "三级故障阀值", "控制参数", "电池信息"}
  T9 = cluster{"电池额定容量(A)":dbl, "使用者":dbl, "电池实际容量(A)":dbl, "车架(牌)号":string, "配置文件版本":string, "SOH(%)":dbl, "SOC(%)":dbl, "产品编号":string, "系统时钟":string}
  T10 = cluster{"总电压过高":dbl, "整组电压不均衡":dbl, "SOC过高":dbl, "单体电压过高":dbl, "总电压过低":dbl, "温度过高":dbl, "温度过低":dbl, "单组电压不均衡":dbl, "整组温度不均衡":dbl, "单组温度不均衡":dbl, "单体电压过低":dbl, "充电电流过高":dbl, "放电电流过高":dbl, "SOC过低":dbl, "内阻过大":dbl, "极柱温度过高":dbl, "SOH过低":dbl}
  T11 = cluster{"风机开启温度":dbl, "风机关闭温度":dbl, "加热开启温度":dbl, "加热关闭温度":dbl, "风机开启温差":dbl, "风机关闭温差":dbl, "加热关闭温差":dbl}
  T12 = cluster{"最大允许单体电压":dbl, "最大允许总电压":dbl, "最小允许单体电压":dbl, "最大允许充电电流":dbl, "最小允许充电电流":dbl, "最大允许充电温度":dbl, "最小允许充电温度":dbl, "电流步长":dbl}
  T13 = cluster{"电池串联":dbl, "电池并联":dbl, "累计放电总安时":dbl, "电池包额定容量":dbl, "电池包额定能量(kWh)":dbl, "电池包额定总电压":dbl, "累计充电总安时":dbl, "电池充满次数":dbl, "电池放空次数":dbl, "电池充电次数":dbl, "电池生产日期":string, "电池厂家":string, "电池类型":string, "电池包组号":string, "电池包产权标识":string, "电池应用车型":string, "实际容量":dbl}
  T14 = enum32{"从板信息", "一级故障阀值", "二级故障阀值", "三级故障阀值", "快换参数", "均衡参数"}
  T15 = cluster{"电压过高":dbl, "电压过低":dbl, "温度过高":dbl, "温度过低":dbl, "电压不均衡(V)":dbl, "温度不均衡":dbl, "SOC过低":dbl}
  T16 = cluster{"串联数":dbl, "并联数":dbl, "电池厂家":dbl, "电池类型":dbl, "额定能量":dbl, "额定容量":dbl, "实际容量":dbl, "额定总压":dbl, "产权标识":dbl, "应用车型":dbl, "电池包组号":dbl, "SOC":dbl, "充电总安时":dbl, "放电总安时":dbl, "放空次数":dbl, "充满次数":dbl, "充电次数":dbl, "车牌号":string, "生产日期":string, "最大允许单体电压":dbl, "最大允许总电压":dbl, "最大允许温度":dbl, "最小允许温度":dbl, "最大允许充电电流":dbl, "最小允许充电电流":dbl, "最小允许单体电压":dbl, "电流步长":dbl, "电池包序号":dbl}
  T17 = cluster{"充电结束电压(90%)":sgl, "充电结束电压(91%)":sgl, "充电结束电压(92%)":sgl, "充电结束电压(93%)":sgl, "充电结束电压(94%)":sgl, "均衡计算-电压高阀值1级":sgl, "均衡计算-电压高阀值2级":sgl, "均衡计算-电压低阀值1级":sgl, "均衡计算-电压低阀值2级":sgl, "均衡计算-最低电压阀值":sgl, "均衡停止-最低电压阀值":sgl, "均衡计算-电压极差阀值":sgl, "充电结束电压(95%)":sgl, "充电结束电压(96%)":sgl, "充电结束电压(97%)":sgl, "充电结束电压(98%)":sgl, "充电结束电压(99%)":sgl, "充电结束电压(100%)":sgl}
  T18 = enum16{"电压,内总电压,外总电压,温度,电流,绝缘,系统时钟,充电均衡,放电均衡", "CPU,CPU内部EE存储器,CPU内部FLASH,内部EE存储器,45db存储器", "CAN检测故障", "软件故障", "RS485,RS232检测故障", "DI,DO,AI,AO检测故障", "预充电故障,继电器驱动故障"}
  T19 = typedef "NI_LVConfig.lvlib/Config Data RefNum.ctl" = refnum<k1>
  T20 = cluster{"[0]":dbl, "[1]":dbl, "[2]":dbl, "[3]":dbl, "[4]":dbl, "[5]":dbl, "[6]":dbl}
  T21 = enum32{"从板信息", "一级故障阀值", "二级故障阀值", "三级故障阀值", "快换参数"}
  T22 = cluster{"fiter_mode":u32, "fiter_endid":u32, "fiter_startid":u32}
  T23 = cluster{"打开CAN":bool, "初始化CAN":bool, "开始CAN":bool, "重启":bool, "关闭CAN":bool}
  T24 = enum32{"Invalid", "Standard", "Closed", "Hidden", "Minimized", "Maximized"}
  T25 = cluster{"return type":u32, "pReceive":cluster{"ID":u32, "TimeStamp":u32, "TimeFlag":u8, "SendType":u8, "RemoteFlag":u8, "ExternFlag":u8, "DataLen":u8, "1":u8, "2":u8, "3":u8, "4":u8, "5":u8, "6":u8, "7":u8, "8":u8, "9":u8, "10":u8, "11":u8}[]}
  T26 = cluster{"ID":u32, "TimeStamp":u32, "TimeFlag":u8, "SendType":u8, "RemoteFlag":u8, "ExternFlag":u8, "DataLen":u8, u8, u8, u8, u8, u8, u8, u8, u8, u8, u8, u8}[]
  T27 = cluster{"电池额定容量":dbl, "使用者":dbl, "电池实际容量":dbl, "车牌号":string, "配置文件版本":string, "SOH":dbl, "SOC":dbl, "产品编号":string, "系统时钟":string}
  T28 = cluster{"电池串联":dbl, "电池并联":dbl, "累计放电总安时":dbl, "电池包额定容量":dbl, "电池包额定能量":dbl, "电池包额定总电压":dbl, "累计充电总安时":dbl, "电池充满次数":dbl, "电池放空次数":dbl, "电池充电次数":dbl, "电池生产日期":string, "电池厂家":string, "电池类型":string, "电池包组号":string, "电池包产权标识":string, "电池应用车型":string, "实际容量":dbl}
  T29 = cluster{"电池类型":dbl, "电池厂家":dbl, "电池地区":dbl, "电池组序号":dbl, "电池包串联数":dbl, "电池包并联数":dbl, "电池包安时数":dbl, "电池包序号":dbl, "充电次数":dbl, "充满电时间":dbl, "放空时间":dbl, "车牌号":string, "最大允许单体电压":dbl, "最大允许总电压":dbl, "最大允许温度":dbl, "最小允许温度":dbl, "最大允许充电电流":dbl, "最小允许充电电流":dbl, "最小允许单体电压":dbl, "电流步长":dbl, "SOC":dbl, "充电总安时":dbl, "放电总这时":dbl}
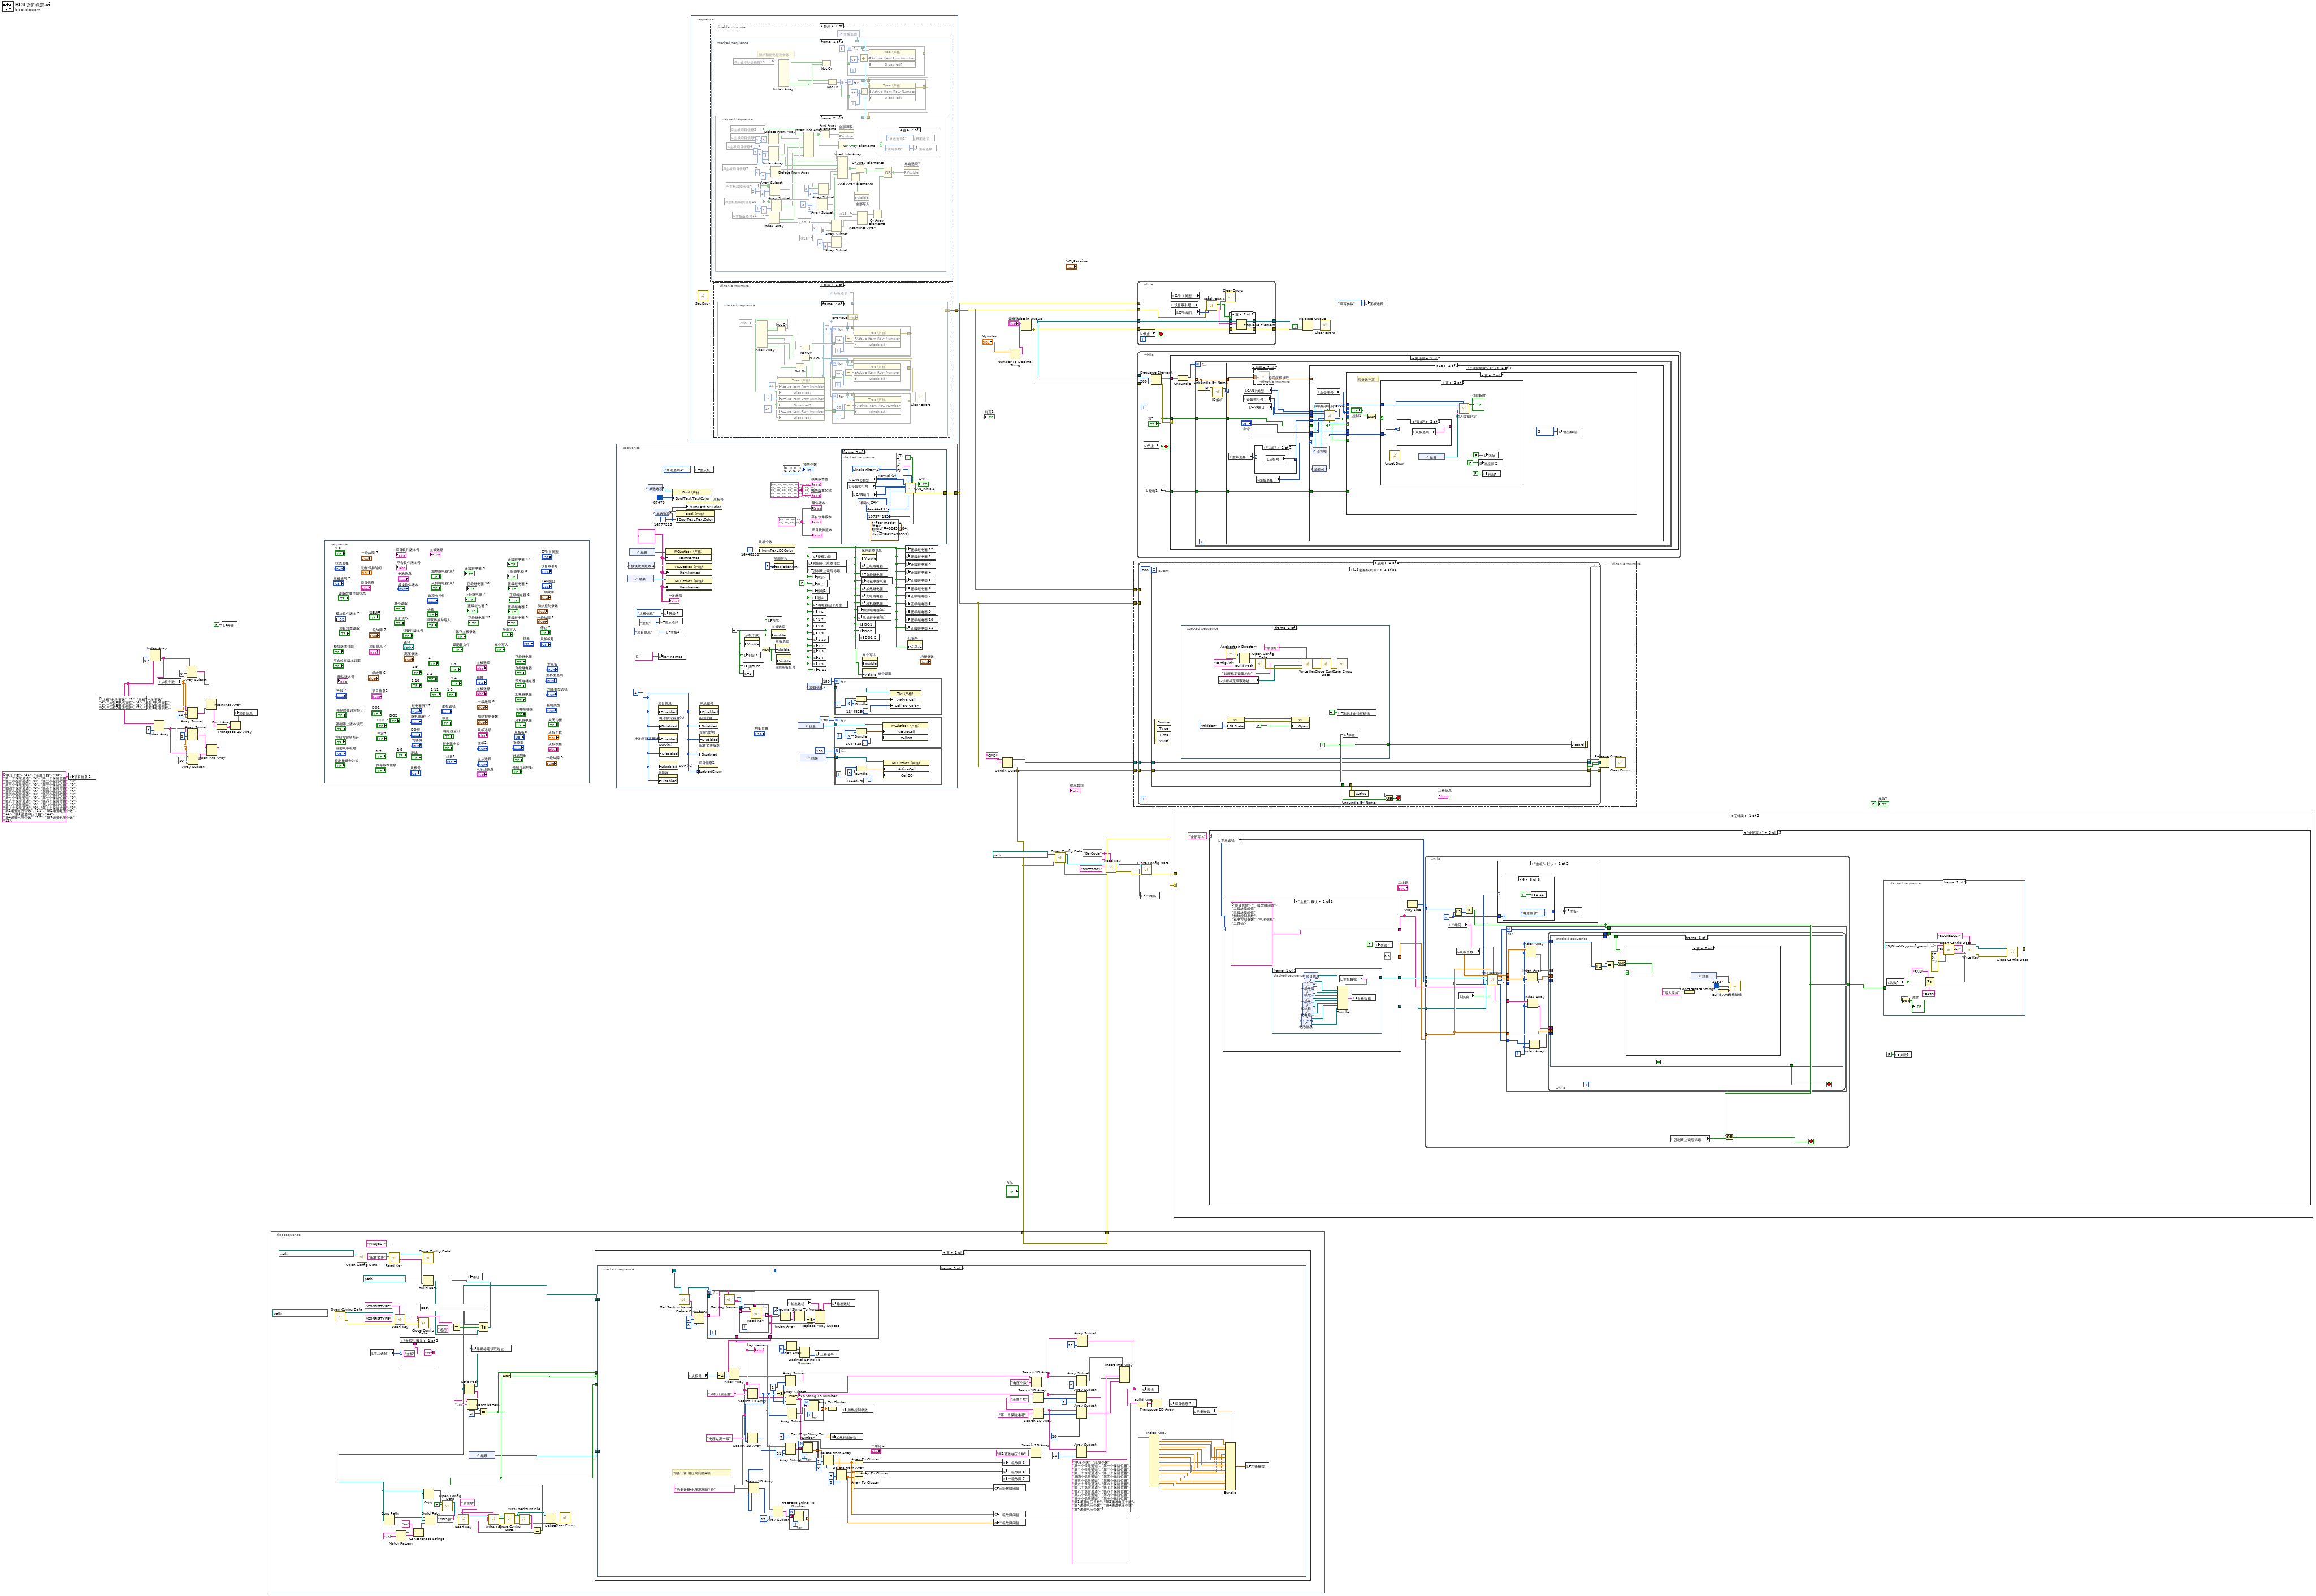
[diagram p0: block diagram]
diagram:
  w11 = "BarCode" ("section")
  w27 = string[][] [["从板1电池节数", "1"], ["从板2电池节数", "2"], ["从板3电池节数", "3"], ["从板4电池节数", "4"], ["从板5电池节数", "5"], ["从板6电池节数", "6"], ["从板7电池节数", "7"], ["从板8电池节数", "8"], ["从板9电池节数", "9"], ["从板10电池节数", "10"], ["从板1温度个数", "1"], ["从板2温度个数", "2"], ["从板3温度个数", "3"], ["从板4温度个数", "4"], ["从板5温度个数", "5"], ["从板6温度个数", "6"], ["从板7温度个数", "7"], ["从板8温度个数", "8"], ["从板9温度个数", "9"], ["从板10温度个数", "10"]] ("项目信息")
  w46 = "CMD" ("名称（未命名）")
  n1 = local write "项目信息 2"(string[][] [["电压个数", "36"], ["温度个数", "45"], ["第一个保险通道", "0"], ["第一个保险位置", "0"], ["第二个保险通道", "0"], ["第二个保险位置", "0"], ["第三个保险通道", "0"], ["第三个保险位置", "0"], ["第四个保险通道", "0"], ["第四个保险位置", "0"], ["第五个保险通道", "0"], ["第五个保险位置", "0"], ["第六个保险通道", "0"], ["第六个保险位置", "0"], ["第七个保险通道", "0"], ["第七个保险位置", "0"], ["第八个保险通道", "0"], ["第八个保险位置", "0"], ["第九个保险通道", "0"], ["第九个保险位置", "0"], ["第十个保险通道", "0"], ["第十个保险位置", "0"], ["第1通道电压个数", "11"], ["第2通道电压个数", "12"], ["第3通道电压个数", "12"], ["第4通道电压个数", "12"], ["第5通道电压个数", "12"]] ("项目信息 2")) -> ()
  n2 = Index Array(array=w27, index (col)=0 ("索引 (行)")) -> (element=w30:string[])  [unwired: 1 in]
  n3 = Index Array(array=w27, index (col)=1 ("禁用的索引 (列)")) -> (element=w20:string[])  [unwired: 1 in]
  n4 = local read "从板个数"() -> (w22:dbl)
  n5 = Array Subset(array=w30, index=0 ("索引"), length=w22) -> (w29:string[])
  n6 = Array Subset(array=w30, index=10 ("索引"), length=w22) -> (w28:string[])
  n7 = Array Subset(array=w20, index=0 ("索引"), length=w22) -> (w26:string[])
  n8 = Array Subset(array=w20, index=10 ("索引"), length=w22) -> (w21:string[])
  n9 = Insert Into Array(array=w29, new element=w28) -> (w19:string[])  [unwired: 1 in]
  n10 = Insert Into Array(array=w26, new element=w21) -> (w18:string[])  [unwired: 1 in]
  n11 = Build Array(w19, w18) -> (w17:string[][])
  n12 = local write "停止"(FALSE ("停止")) -> ()
  n13 = Transpose 2D Array(2D array=w17) -> (transposed array=w16:string[][])
  n14 = local write "项目信息"(w16) -> ()
  n15 = flat-sequence {
    tunnel: w8 -> [w60]
    tunnel: [w60] -> w14
    frame #0 {
      w86 = "MD5码" ("key")
      w87 = "总信息" ("section")
      n16 = call <vilib>:"Open Config Data.vi"("configuration file path"=path "D:/BlueWay/BMU从板号.ini") -> ("error out"=w53:errorcluster, "refnum"=w54:T19)  [unwired: 8 in, 1 out]
      n17 = call <vilib>:"Open Config Data.vi"("configuration file path"=path "D:/自动测试项目文件/ProjectSetting.ini") -> ("refnum"=w67:T19)  [unwired: 8 in, 2 out]
      n18 = local read "主从选择"() -> (w91:enum32{"主板", "从板"})
      n19 = call-poly <vilib>:"Read Key.vi"("section"="PROJECT", "key"="配置文件", "refnum"=w67) -> ("value"=w62:string, "refnum out"=w66:T19)  [unwired: 5 in, 2 out]
      n20 = call-poly <vilib>:"Read Key.vi"("section"="CONFIGTYPE", "error in (no error)"=w53, "key"="CONFIGTYPE", "refnum"=w54) -> ("error out"=w57:errorcluster, "value"=w50:string, "refnum out"=w56:T19)  [unwired: 4 in, 1 out]
      n21 = case shown="\"主板\", 默认" w91 {
        tunnel: ["M" ("pattern (all files)") "S" ("pattern (all files)")] -> _
        tunnel: ["主板" ("pattern (all files)") "从板" ("pattern (all files)")] -> _
        frame "主板", Default {
        }
        frame "从板" {
        }
      }
      n22 = call <vilib>:"Close Config Data.vi"("error in (no error)"=w57, "refnum"=w56) -> ()  [unwired: 8 in, 2 out]
      n23 = call <vilib>:"Close Config Data.vi"("refnum"=w66) -> ()  [unwired: 9 in, 2 out]
      n24 = Build Path(base path=path "D:/自动测试项目文件" ("configuration file path"), name or relative path=w62) -> (appended path=w49:path)
      n25 = Equal?(x=w50, y="通用") -> (x = y?=w52:bool)
      n26 = control-ref of="结果"() -> (w92:refnum<vi>)
      n27 = Select(t=path "D:/BlueWay/通用文件/通用配置.ini", s=w52, f=w49) -> (s? t:f=w48:path)
      n28 = Strip Path(path=w48) -> (stripped path=w74:path, name=w73:string)
      n29 = Match Pattern(string=w73, regular expression=".ini" ("正则表达式")) -> (before substring=w70:string, match substring=w71:string)  [unwired: 1 in, 2 out]
      n30 = Concatenate Strings(w70, "-rc" ("字符串"), w71) -> (w69:string)
      n31 = Build Path(base path=w74, name or relative path=w69) -> (appended path=w75:path)
      n32 = Copy(10:w75, 11:w48) -> (3:w79:path)  [unwired: 3 in, 2 out]
      n33 = call <vilib>:"Open Config Data.vi"("create file if necessary (T)"=FALSE, "configuration file path"=w79) -> ("refnum"=w89:T19)  [unwired: 7 in, 2 out]
      n34 = call-poly <vilib>:"Read Key.vi"("section"=w87, "key"=w86, "refnum"=w89) -> ("value"=w84:string, "refnum out"=w88:T19)  [unwired: 5 in, 2 out]
      n35 = Strip Path(path=w48) -> (stripped path=w100:path, name=w93:string)
      n36 = local write "路径"(w48) -> ()
      n37 = Match Pattern(string=w93, regular expression=".ini" ("正则表达式")) -> (offset past match=w95:i32)  [unwired: 1 in, 3 out]
      n38 = global write "配置文件全局.vi" "诊断标定读取地址"(w100) -> ()
      n39 = Not Equal?(x=w95, y=-1) -> (x != y?=w99:bool)
      n40 = call-poly <vilib>:"Write Key.vi"("section"=w87, "value"=w86, "key"=w86, "refnum"=w88) -> ("error out"=w83:errorcluster, "found?"=w82:bool, "refnum out"=w81:T19)  [unwired: 5 in]
      n41 = call <vilib>:"Close Config Data.vi"("error in (no error)"=w83, "write file if changed (T)"=w82, "refnum"=w81) -> ("error out"=w80:errorcluster, "file path"=w77:path)  [unwired: 7 in]
      n42 = call <vilib>:"MD5Checksum File.vi"("error in (no error)"=w80, "Path"=w77) -> ("error out"=w78:errorcluster, "MD5 message-digest"=w85:string)  [unwired: 8 in]
      n43 = Equal?(x=w85, y=w84) -> (x = y?=w98:bool)
      n44 = And(x=w99, y=w98) -> (x .and. y?=w97:bool)
      n45 = Delete(path (use dialog)=w77, error in=w78) -> (error out=w76:errorcluster)  [unwired: 3 in, 2 out]
      n46 = call <vilib>:"Clear Errors.vi"("error in (no error)"=w76) -> ()  [unwired: 6 in, 1 out]
      n47 = case shown="真" w97 {
        tunnel: w48 -> [_ w117]
        tunnel: w92 -> [w103 w116]
        tunnel: w98 -> [w102 _]
        tunnel: w99 -> [w101 _]
        frame False {
          n48 = stacked-sequence {
